vi "DB - [Config].[UnitOfMeasurement].vi"(4 "[UnitOfMeasurementId]":string="01", 5 "[LanguageId]":string="EN", 6 "[PlantId]":string="4070", 7 "DB Connection":T2={"Open"=TRUE, "Close"=TRUE}, 8 "error in (no error)":errorcluster, 11 "connection reference":T1) -> (0 "SUMMARY":errorcluster, 1 "Unit Of Measurement":string="°C", 2 "data":string[][](array[string])=[["°C"]], 3 "connection reference":T1)   [LabVIEW 2013]
uses:
  <vilib>/addons/database/Connection.llb/Conn ObjectReference.ctl
  Controls/DB - OpenClose.ctl
  <vilib>/addons/database/Connection.llb/Conn Execute.vi
  <vilib>/addons/database/Recordset.llb/Rec Fetch Recordset Data (R).vi
  <vilib>/addons/database/Recordset.llb/Rec Destroy - Connection.vi
  Controls/Global SRTRS.vi
  <vilib>/addons/database/Connection.llb/DB Tools Open Connec (String).vi
  <vilib>/addons/database/_DB Variant To Data/Database Variant To Data.xnode
  <vilib>/addons/database/NI_Database_API.lvlib
panel:
  out "Close":errorcluster
  out "SQL Statement":string="USE [SRTRS]\nSELECT \n  [Description]\nFROM [Config].[UnitOfMeasurement]\nWHERE\n[PlantId] = '4070' AND\n[LanguageId] = 'EN' AND\n[UnitOfMeasurementId] = '01' AND\n[Inactive] = '0'"
  in  "DB.Schema.Table\nSRTRS.Config.UnitOfMeasurement":string="SRTRS.Config.UnitOfMeasurement"
  out "Connection Information":T3={"Connection "="SQL Server 32bit HPEnvy", "Username"="admin", "Password"="admin123"}
  # "2014-0-28 18:29\n[Furnace Serial No]                        [Eurotherm]                 [Model]                                     [Description]                            [Equipment Serial No]                  [EquipmentId]                [LastCalibDate]                         [NextCalibDate]"
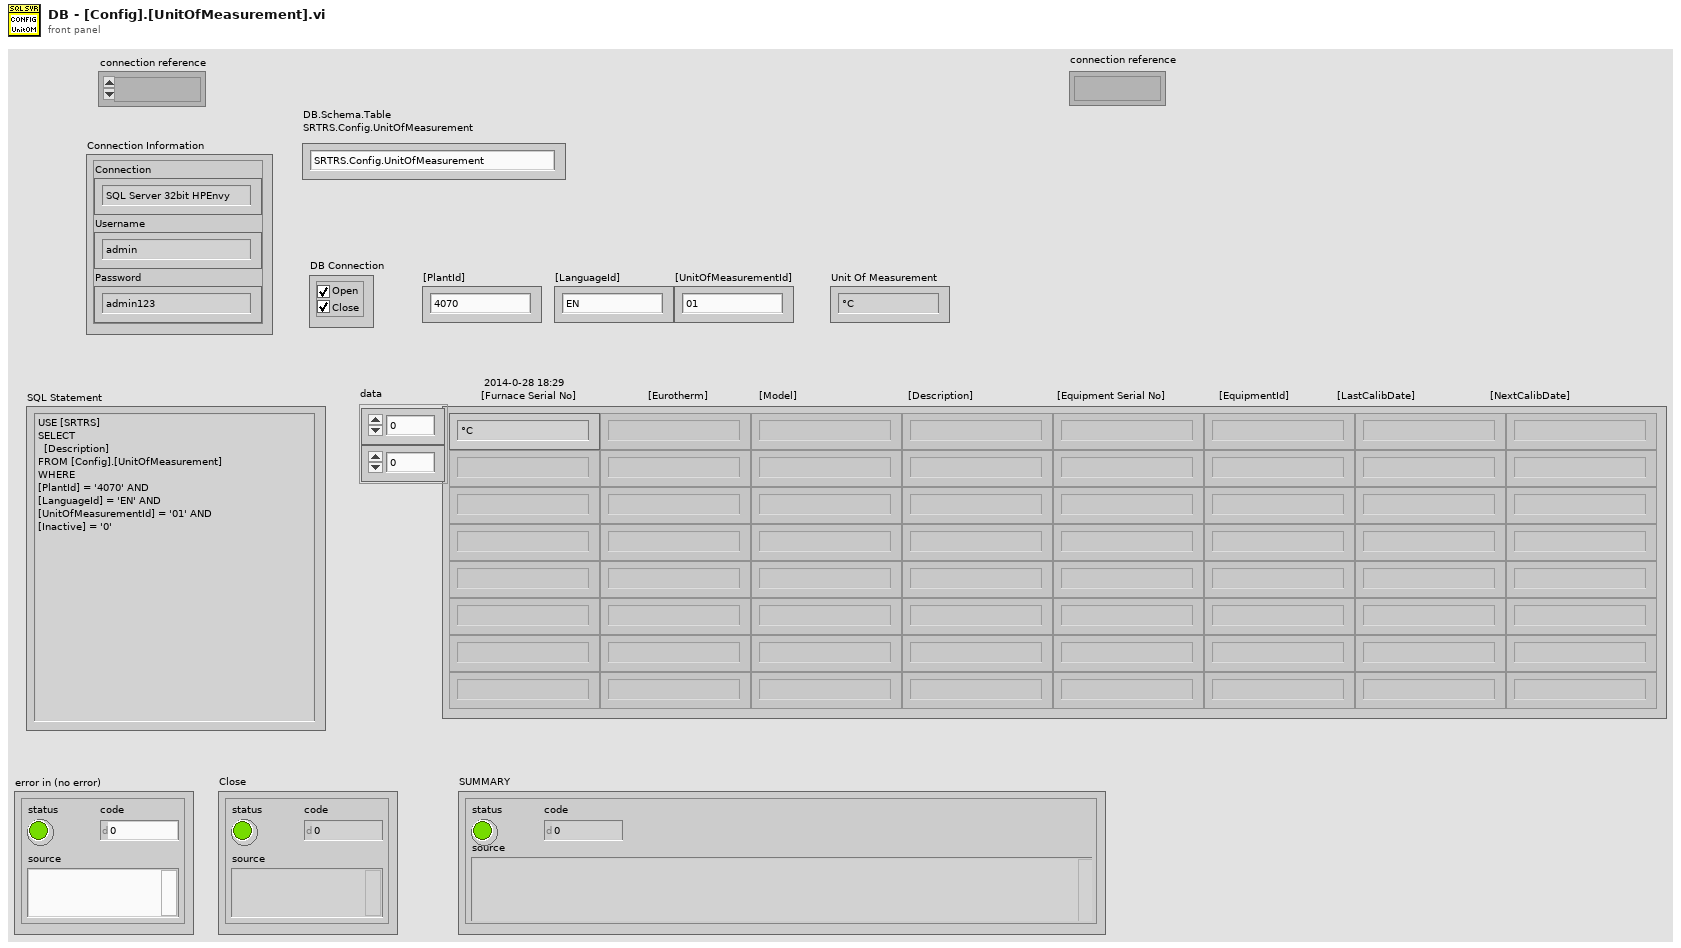
[diagram p1: front panel]
types:
  T1 = typedef "NI_Database_API.lvlib/Conn ObjectReference.ctl" = refnum<k1>
  T2 = typedef "DB - OpenClose.ctl" = cluster{"Open":bool, "Close":bool}
  T3 = cluster{"Connection ":string, "Username":string, "Password":string}
  T4 = typedef "Enum - InteractiveMode-SubVIMode.ctl" = enum16{"Interactive", "subVI Mode"}
  T5 = typedef "DB - DB.Schema.Table.ctl" = cluster{"DB":string, "Schema":string, "Table":string}
  T6 = typedef "Connection Information Cluster.ctl" = cluster{"Connection ":string, "Username":string, "Password":string}
  T7 = typedef "NI_Database_API.lvlib/Rec ObjectReference.ctl" = refnum<k1>
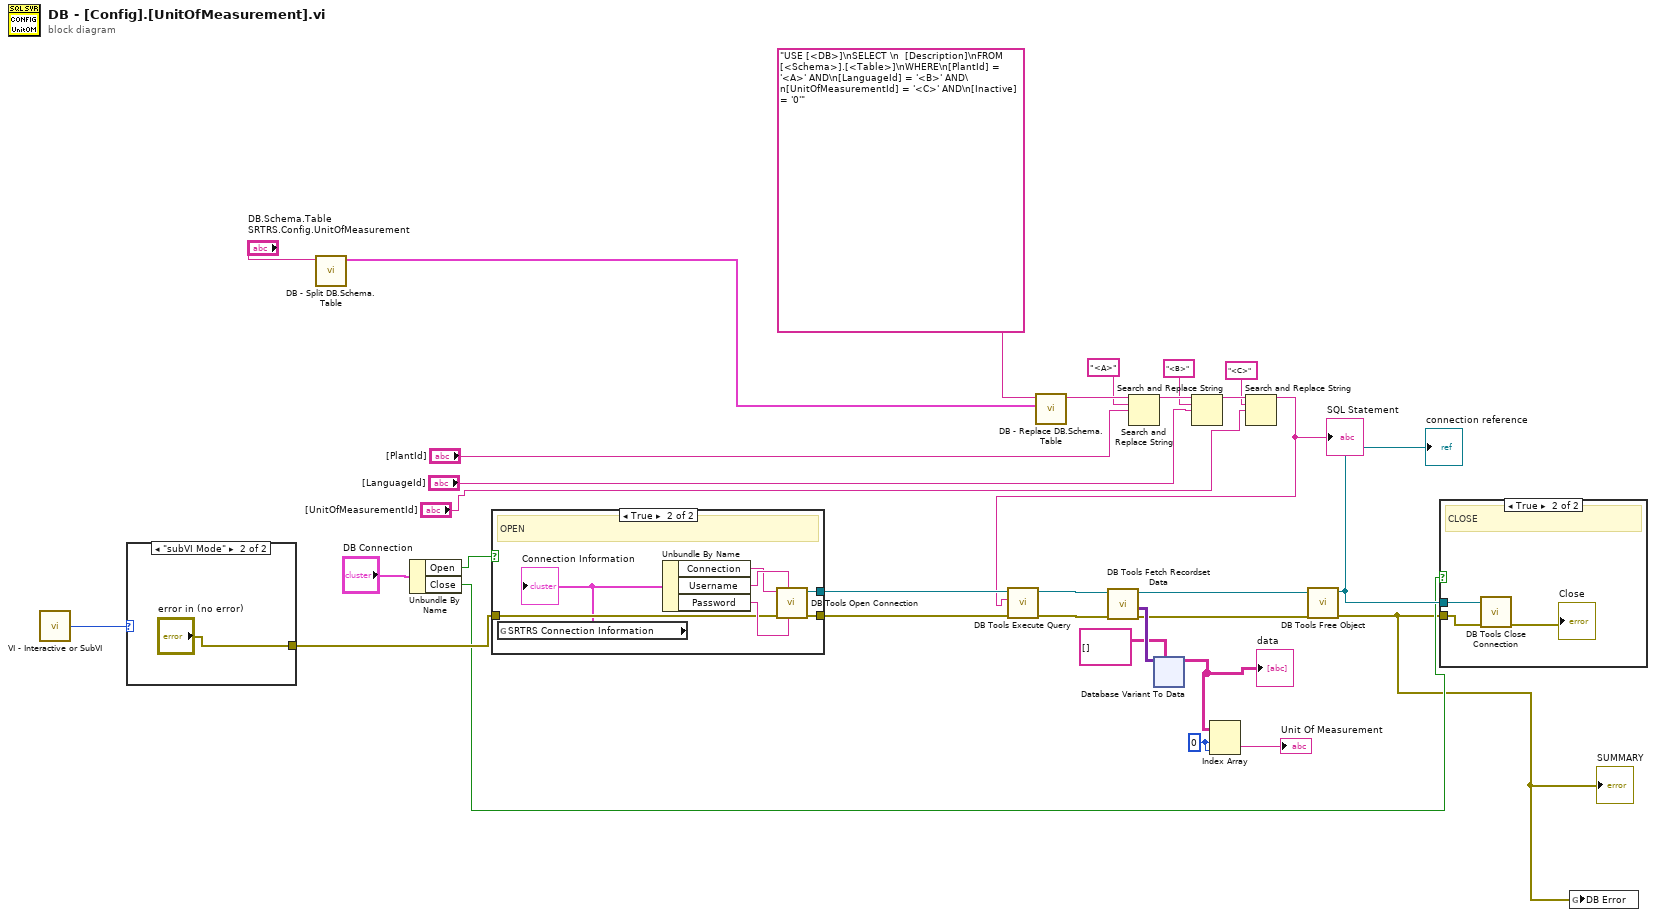
[diagram p0: block diagram]
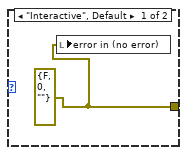
[diagram p3: hidden frame]
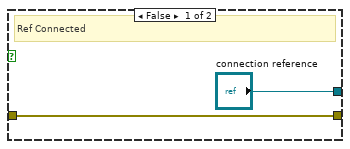
[diagram p4: hidden frame]
diagram:
  w2 = 0 ("index (row)")
  n1 = call "VI - Interactive or SubVI.vi"() -> ("Mode"=w29:T4)  [unwired: 5 in]
  n2 = case shown="\"subVI Mode\"" w29 {
    tunnel: [w32 "error in (no error)"] -> w28
    frame "Interactive", Default {
      w32 = errorcluster {"status"=FALSE, "code"=0, "source"=""} ("error in (no error)")
      n3 = local write "error in (no error)"(w32) -> ()
    }
    frame "subVI Mode" {
    }
  }
  n4 = call "DB - Split DB.Schema.Table.vi"("DB.Schema.Table"="DB.Schema.Table\nSRTRS.Config.UnitOfMeasurement") -> ("DB.Schema.Table"=w16:T5)  [unwired: 10 in]
  n5 = Unbundle By Name("DB Connection") -> ("Open"=w30:bool, "Close"=w18:bool)
  n6 = case shown="True" w30 {
    tunnel: ["connection reference" w39] -> w21
    tunnel: w28 -> [w34 w38]
    tunnel: [w34 w37] -> w20
    frame False {
      # "Ref Connected"
    }
    frame True {
      # "OPEN"
      n7 = global read "Global SRTRS.vi" "SRTRS Connection Information"() -> (w36:T6)
      "Connection Information" <- w36
      n8 = Unbundle By Name(w36) -> ("Connection"=w41:string, "Username"=w42:string, "Password"=w40:string)
      n9 = call-poly <vilib>:"DB Tools Open Connection.vi"("password"=w40, "userID"=w42, "error in (no error)"=w38, "connection information"=w41) -> ("error out"=w37:errorcluster, "connection reference"=w39:T1)  [unwired: 4 in]
    }
  }
  n10 = call "DB - Replace DB.Schema.Table.vi"("DB.Schema.Table"=w16, "string in"="USE [<DB>]\nSELECT \n  [Description]\nFROM [<Schema>].[<Table>]\nWHERE\n[PlantId] = '<A>' AND\n[LanguageId] = '<B>' AND\n[UnitOfMeasurementId] = '<C>' AND\n[Inactive] = '0'") -> ("string out"=w14:string)  [unwired: 8 in, 1 out]
  n11 = Search and Replace String(input string=w14, search string="<A>", replace string="[PlantId]") -> (result string=w11:string)  [unwired: 5 in, 3 out]
  n12 = Search and Replace String(input string=w11, search string="<B>", replace string="[LanguageId]") -> (result string=w7:string)  [unwired: 5 in, 3 out]
  n13 = Search and Replace String(input string=w7, search string="<C>", replace string="[UnitOfMeasurementId]") -> (result string=w6:string)  [unwired: 5 in, 3 out]
  "SQL Statement" <- w6
  n14 = call-poly <vilib>:"DB Tools Execute Query.vi"("error in (no error)"=w20, "SQL query"=w6, "connection reference"=w21) -> ("error out"=w27:errorcluster, "recordset reference"=w26:T7)  [unwired: 5 in]
  n15 = call-poly <vilib>:"DB Tools Fetch Recordset Data.vi"("error in (no error)"=w27, "recordset reference"=w26) -> ("error out"=w22:errorcluster, "recordset data"=w25:variant[][], "recordset reference out"=w23:T7)  [unwired: 3 in]
  n16 = xnode "Database Variant To Data"("database variant"=w25, "type"=string[][] []) -> ("data"=w3:string[][])  [unwired: 1 in, 1 out]
  "data" <- w3
  n17 = Index Array(array=w3, index (row)=w2, index (col)=w2) -> (element=→"Unit Of Measurement":string)
  n18 = call-poly <vilib>:"DB Tools Free Object.vi"("error in (no error)"=w22, "recordset reference"=w23) -> ("error out"=w8:errorcluster, "connection reference"=w19:T1)  [unwired: 8 in]
  "SUMMARY" <- w8
  "connection reference" <- w19
  n19 = case shown="True" w18 {
    tunnel: w19 -> [_ w45]
    tunnel: w8 -> [_ w44]
    frame False {
      # "Ref Connected"
    }
    frame True {
      # "CLOSE"
      n20 = call <vilib>:"DB Tools Close Connection.vi"("error in (no error)"=w44, "connection reference"=w45) -> ("error out"=→"Close":errorcluster)  [unwired: 5 in]
    }
  }
  n21 = global write "Global SRTRS.vi" "DB Error"(w8) -> ()
